vi "FGV ARN Protokoll.vi"(6 "Aktion":T2, 8 "error in (no error)":errorcluster caption="Fehler (Eingang, kein Fehler)", 10 "ResultPictures":T1, 11 "SVGraph Referenz":refnum<vi>) -> (0 "error out":errorcluster caption="Fehler (Ausgang)", 2 "Tabelle Wertänderung":bool, 3 "Tabelle":string[][](array[string]))   [LabVIEW 2020, in "EPA 1065.lvlib" / "ARN Test 1065-305.lvlib"]
uses:
  ARN Test 1065-305.lvlib
  Aktion FGV ARN Protokoll.ctl
  PDF_Interface/PDF Interface Helper/PDFResultPictures.ctl
  Seiten/Gaszuordnung AO/FGV Gaszuordnung Grenzen&Einheit Aktion.ctl
  Aktion FGV ARN Daten.ctl
  Seiten/FT-IR/FGV FT-IR Gasliste Aktionen.ctl
  Sprachverwaltung/FGV Aktion Tabelle zerlegen.ctl
  Cluster PDF.ctl
  Visualisierungs Elemente/String - Ausgabefeld.ctl
  Aktion FGV Protokoll.ctl
  Seiten/Gaszuordnung AO/Gaszuordnung AO.lvlib
  Sprachverwaltung/Sprachverwaltung.lvlib
  Seiten/FT-IR/FT-IR.lvlib
  Linearisierung V2/EPA1065-307/Linearity verification 1065-307.lvlib
  Linearisierung V2/Protokoll/Protokoll.lvlib
  PDF_Interface/PDF Interface Helper/PDF Interface Helper.lvlib
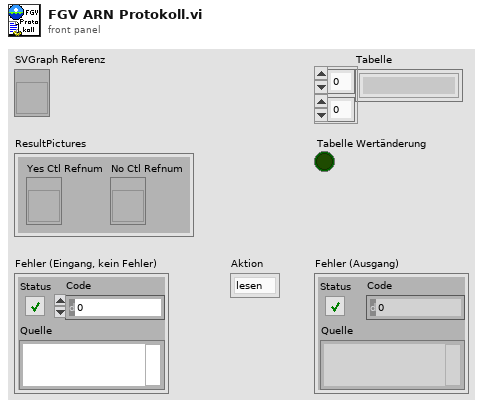
[diagram p1: front panel]
types:
  T1 = typedef "PDF Interface.lvlib/PDF Interface Helper.lvlib/PDFResultPictures.ctl" = cluster{"Yes Ctl Refnum":refnum<vi>, "No Ctl Refnum":refnum<vi>}
  T2 = typedef "EPA 1065.lvlib/ARN Test 1065-305.lvlib/Aktion FGV ARN Protokoll.ctl" = enum16{"lesen", "Tab. schreiben", "Protokoll ausw.", "Protokoll speichern", "Textdatei speichern"}
  T3 = typedef "FT-IR.lvlib/FGV FT-IR Gasliste Aktionen.ctl" = enum16{"lesen", "Gasliste FT-IR", "Gasliste ausgelesen", "laden", "speichern", "löschen"}
  T4 = typedef "EPA 1065.lvlib/ARN Test 1065-305.lvlib/Aktion FGV ARN Daten.ctl" = enum16{"Lesen", "laden", "speichern", "ARN Daten", "Rohdaten", "Rohdaten löschen", "Zeitstempel", "SNR Ergebnis"}
  T5 = typedef "Gaszuordnung AO.lvlib/FGV Gaszuordnung Grenzen&Einheit Aktion.ctl" = enum16{"Lesen", "Schreiben Min", "Schreiben Max", "Laden", "Speichern"}
  T6 = typedef "EPA 1065.lvlib/ARN Test 1065-305.lvlib/Aktion FGV Protokoll.ctl" = enum16{"lesen", "schreiben", "Graph"}
  T7 = typedef "EPA 1065.lvlib/ARN Test 1065-305.lvlib/Cluster PDF.ctl" = cluster{"TAB 1":T8[][], "TAB 2":string[][], "TAB 3":string[][], "Error":bool[]}
  T8 = typedef "String - Ausgabefeld.ctl" = string
  T9 = typedef "Sprachverwaltung.lvlib/FGV Aktion Tabelle zerlegen.ctl" = enum16{"laden", "vereinzeln", "speichern"}
  T10 = enum16{"open", "replace", "create", "open or create", "replace or create", "replace or create with confirmation"}
  T11 = typedef "EPA 1065.lvlib/ARN Test 1065-305.lvlib/Allgemeine Einstellungen.ctl" = cluster{"Bearbeiter:":string, "Analysator":T12, "Komponente:":u16, "Gasflaschen Nr.:":string, "Accuracy":dbl, "Sollwert":dbl, "Modus":T13, "Pfad:":path, "Textname:":string, "CG Aufschaltzeit:":dbl, "Einheit":string, "N2 Aufschaltzeit:":dbl, "Gasflasche":T14, "Konfig Gasflasche":T15}
  T12 = typedef "System Einstellungen V2.lvlib/Analysatoren.ctl" = string
  T13 = typedef "EPA 1065.lvlib/T90 Test 1065-308.lvlib/Modus.ctl" = u16
  T14 = typedef "System Einstellungen V2.lvlib/Gasflasche Auswahl.ctl" = u16
  T15 = typedef "System Einstellungen V2.lvlib/Konfig Gasflasche.ctl" = bool
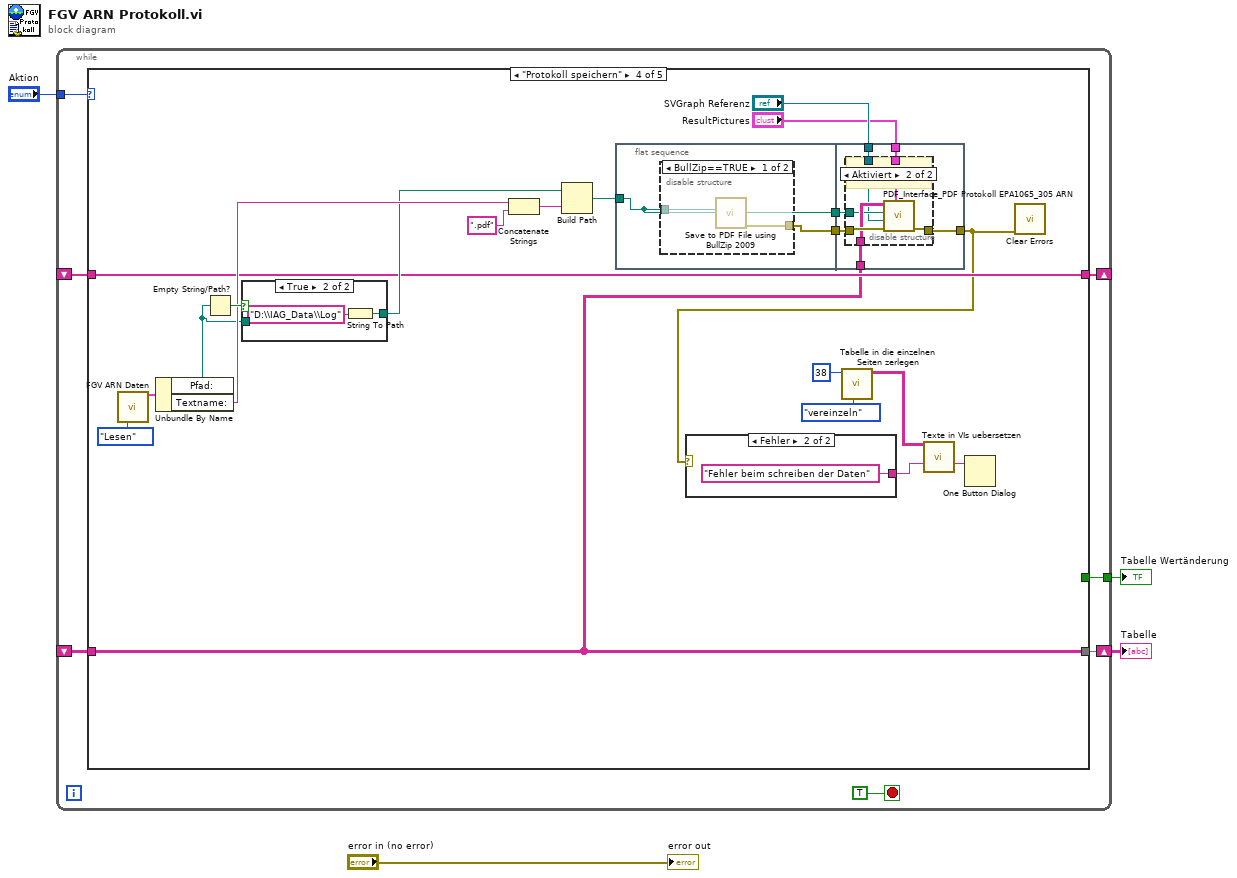
[diagram p0: block diagram]
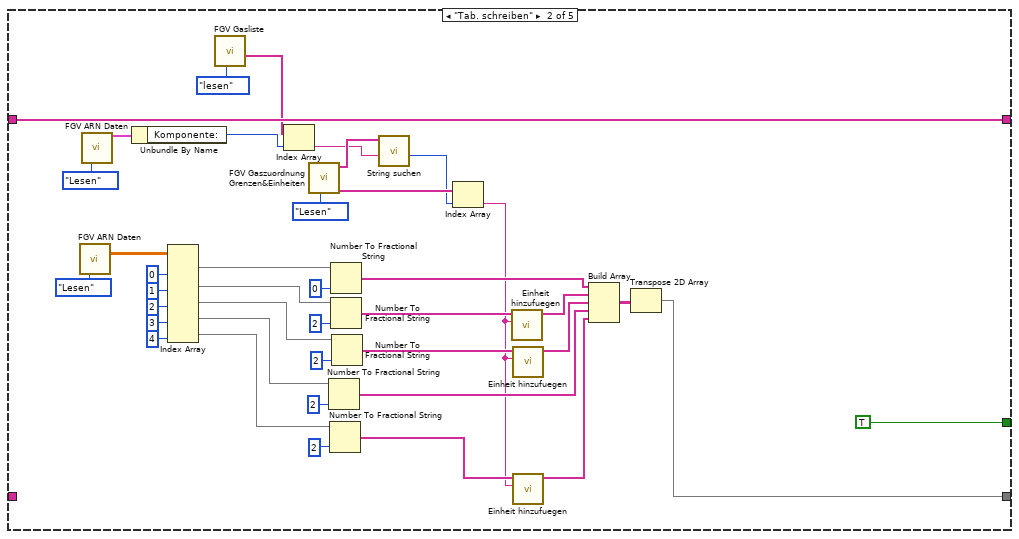
[diagram p3: hidden frame]
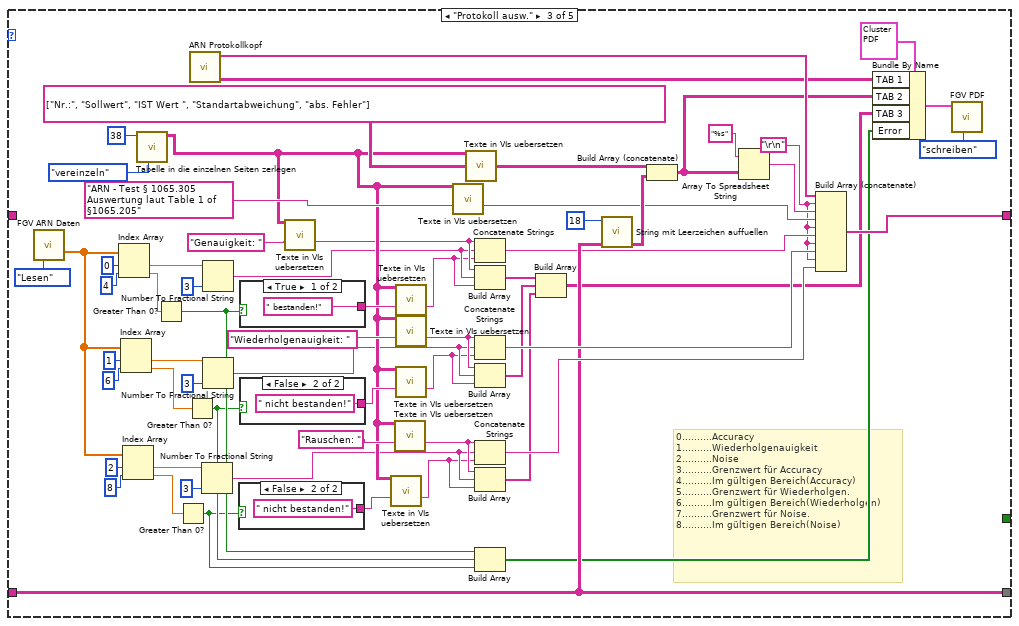
[diagram p4: hidden frame]
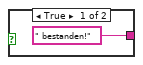
[diagram p5: hidden frame]
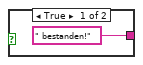
[diagram p6: hidden frame]
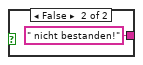
[diagram p7: hidden frame]
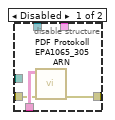
[diagram p9: hidden frame]
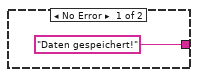
[diagram p11: hidden frame]
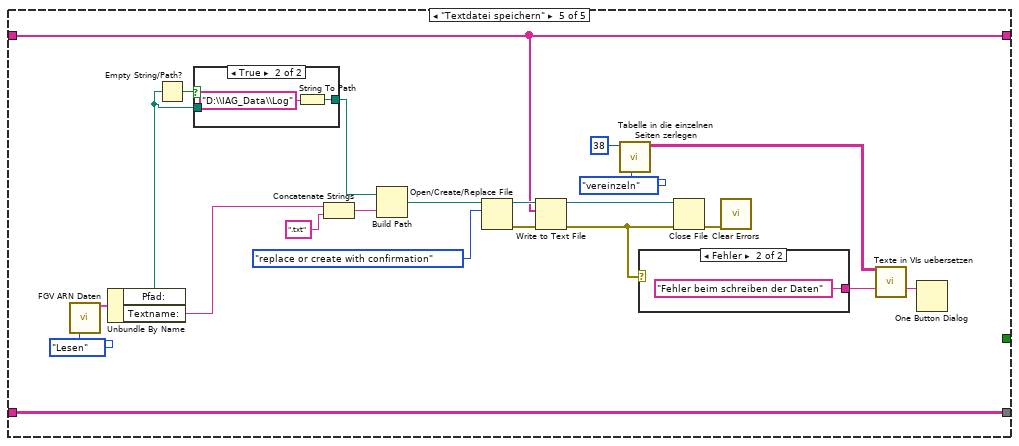
[diagram p12: hidden frame]
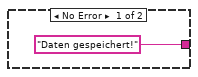
[diagram p14: hidden frame]
diagram:
  n1 = while {
    tunnel: "Aktion" -> [w10]
    shift-right: [w9] -> w3
    shift-left: _ -> [w8]
    shift-right: [w7] -> _
    shift-left: _ -> [w6]
    tunnel: [w5] -> w1
    stop <- TRUE stop-if-true
    n2 = case shown="\"Protokoll speichern\"" w10 {
      tunnel: [w13 w15 w93 w128 w189] -> w9
      tunnel: w8 -> [w13 _ w93 w128 w189]
      tunnel: [w12 w35 w113 w129 w168] -> w7
      tunnel: w6 -> [w12 w35 _ w129 w168]
      tunnel: [_ TRUE _ _ _] -> w5
      frame "lesen", Default {
      }
      frame "Tab. schreiben" {
        n3 = call "FGV ARN Daten.vi"("Aktion"=Aktion_FGV_ARN_Daten."Lesen") -> ("Rohdaten"=w41:sgl[][])  [unwired: 9 in, 5 out]
        n4 = call "FGV ARN Daten.vi"("Aktion"=Aktion_FGV_ARN_Daten."Lesen") -> ("ARN Konfig Daten"=w32:T11)  [unwired: 9 in, 5 out]
        n5 = Unbundle By Name(w32) -> ("Komponente:"=w19:u16)
        n6 = Index Array(array=w41, index (col) #1=0 ("Deaktivierter Index (Spalte)"), index (col) #2=1 ("Index (Spalte)"), index (col) #3=2 ("Index (Spalte)"), index (col) #4=3 ("Index (Spalte)"), index (col) #5=4 ("Index (Spalte)")) -> (element #1=w51:sgl[], element #2=w50:sgl[], element #3=w48:sgl[], element #4=w46:sgl[], element #5=w42:sgl[])  [unwired: 5 in]
        n7 = call "FGV Gasliste.vi"("Aktionen"=FGV_FT-IR_Gasliste_Aktionen."lesen") -> ("Aktuelle Gasliste gesamt"=w20:T8[])  [unwired: 8 in, 2 out]
        n8 = Index Array(array=w20, index=w19) -> (element=w17:T8)
        n9 = call "FGV Gaszuordnung Grenzen&Einheiten.vi"("Aktion"=FGV_Gaszuordnung_Grenzen&Einheit_Aktion."Lesen") -> ("Einheit neu"=w31:string[], "Namen neu"=w18:string[])  [unwired: 2 in, 7 out]
        n10 = Number To Fractional String(number=w46, precision (6)=i16 2 ("Genauigkeit (6)")) -> (F-format string=w29:string[])  [unwired: 2 in]
        n11 = Number To Fractional String(number=w42, precision (6)=i16 2 ("Genauigkeit (6)")) -> (F-format string=w24:string[])  [unwired: 2 in]
        n12 = Number To Fractional String(number=w51, precision (6)=i16 0 ("Genauigkeit (6)")) -> (F-format string=w30:string[])  [unwired: 2 in]
        n13 = Number To Fractional String(number=w50, precision (6)=i16 2 ("Genauigkeit (6)")) -> (F-format string=w28:string[])  [unwired: 2 in]
        n14 = Number To Fractional String(number=w48, precision (6)=i16 2 ("Genauigkeit (6)")) -> (F-format string=w26:string[])  [unwired: 2 in]
        n15 = call "String suchen.vi"("Gasname"=w17, "Such-Namen"=w18) -> ("Index"=w16:i32)  [unwired: 8 in, 1 out]
        n16 = Index Array(array=w31, index=w16) -> (element=w22:string)
        n17 = call "Einheit hinzufuegen.vi"("Einheit"=w22, "Eingang"=w28) -> ("Ausgang"=w27:string[])  [unwired: 9 in]
        n18 = call "Einheit hinzufuegen.vi"("Einheit"=w22, "Eingang"=w26) -> ("Ausgang"=w25:string[])  [unwired: 9 in]
        n19 = call "Einheit hinzufuegen.vi"("Einheit"=w22, "Eingang"=w24) -> ("Ausgang"=w23:string[])  [unwired: 9 in]
        n20 = Build Array(w30, w27, w25, w29, w23) -> (w45:string[][])
        n21 = Transpose 2D Array(2D array=w45) -> (transposed array=w15:string[][])
      }
      frame "Protokoll ausw." {
        w54 = "\r\n"
        # "0..........Accuracy\n1..........Wiederholgenauigkeit\n2..........Noise\n3..........Grenzwert für Accuracy\n4..........Im gültigen Bereich(Accuracy)\n5..........Grenzwert für Wiederholgen.\n6..........Im gültigen Bereich(Wiederholgen)\n7..........Grenzwert für Noise.\n8..........Im gültigen Bereich(Noise)"
        n22 = call "FGV ARN Daten.vi"("Aktion"=Aktion_FGV_ARN_Daten."Lesen") -> ("SNR Ergebnis"=w98:sgl[])  [unwired: 9 in, 5 out]
        n23 = Index Array(array=w98, index #1=0 ("Index"), index #2=4 ("Index")) -> (element #1=w111:sgl, element #2=w108:sgl)
        n24 = Index Array(array=w98, index #1=1 ("Index"), index #2=6 ("Index")) -> (element #1=w101:sgl, element #2=w102:sgl)
        n25 = Index Array(array=w98, index #1=2 ("Index"), index #2=8 ("Index")) -> (element #1=w97:sgl, element #2=w96:sgl)
        n26 = call "Tabelle in die einzelnen Seiten zerlegen.vi"("Aktion"=FGV_Aktion_Tabelle_zerlegen."vereinzeln", "Index (Seite)"=38) -> ("Sprachliste"=w80:string[][])  [unwired: 7 in, 2 out]
        n27 = Greater Than 0?(x=w108) -> (x > 0?=w65:bool)
        n28 = Greater Than 0?(x=w96) -> (x > 0?=w63:bool)
        n29 = Greater Than 0?(x=w102) -> (x > 0?=w64:bool)
        n30 = call "ARN Protokollkopf.vi"() -> ("Angehängtes Array"=w62:T8[][], "Kopfzeile"=w115:string[])  [unwired: 10 in]
        n31 = Number To Fractional String(number=w97, precision (6)=i16 3 ("Genauigkeit (6)")) -> (F-format string=w70:string)  [unwired: 2 in]
        n32 = Number To Fractional String(number=w111, precision (6)=i16 3 ("Genauigkeit (6)")) -> (F-format string=w76:string)  [unwired: 2 in]
        n33 = Number To Fractional String(number=w101, precision (6)=i16 3 ("Genauigkeit (6)")) -> (F-format string=w73:string)  [unwired: 2 in]
        n34 = case shown="False" w63 {
          tunnel: [" bestanden!" " nicht bestanden!"] -> w79
          frame True {
          }
          frame False {
          }
        }
        n35 = case shown="True" w65 {
          tunnel: [" bestanden!" " nicht bestanden!"] -> w84
          frame True {
          }
          frame False {
          }
        }
        n36 = case shown="False" w64 {
          tunnel: [" bestanden!" " nicht bestanden!"] -> w82
          frame True {
          }
          frame False {
          }
        }
        n37 = call "Texte in VIs uebersetzen.vi"("Sprachliste"=w80, "String zum Übersetzen"="Genauigkeit: ") -> ("String zum Übersetzen"=w77:string)  [unwired: 9 in, 4 out]
        n38 = call "Texte in VIs uebersetzen.vi"("Sprachliste"=w80, "String zum Übersetzen"=w79) -> ("String zum Übersetzen"=w69:string)  [unwired: 9 in, 4 out]
        n39 = call "Texte in VIs uebersetzen.vi"("Sprachliste"=w80, "String zum Übersetzen"="Rauschen: ") -> ("String zum Übersetzen"=w71:string)  [unwired: 9 in, 4 out]
        n40 = call "Texte in VIs uebersetzen.vi"("Sprachliste"=w80, "String zum Übersetzen"=w84) -> ("String zum Übersetzen"=w75:string)  [unwired: 9 in, 4 out]
        n41 = call "Texte in VIs uebersetzen.vi"("Sprachliste"=w80, "String zum Übersetzen"="Wiederholgenauigkeit: ") -> ("String zum Übersetzen"=w74:string)  [unwired: 9 in, 4 out]
        n42 = call "Texte in VIs uebersetzen.vi"("Sprachliste"=w80, "String zum Übersetzen"=w82) -> ("String zum Übersetzen"=w72:string)  [unwired: 9 in, 4 out]
        n43 = call "Texte in VIs uebersetzen.vi"("Sprachliste"=w80, "String zum Übersetzen"="ARN - Test § 1065.305 Auswertung laut Table 1 of §1065.205") -> ("String zum Übersetzen"=w86:string)  [unwired: 9 in, 4 out]
        n44 = call "Texte in VIs uebersetzen.vi"("Sprachliste"=w80, "2D String-Array zum Übersetzen"=string[][] [["Nr.:", "Sollwert", "IST Wert ", "Standartabweichung", "abs. Fehler"]]) -> ("2D String-Array zum Übersetzen"=w88:string[][])  [unwired: 9 in, 4 out]
        n45 = Concatenate Strings(w77, w76, w75) -> (w55:string)
        n46 = Build Array(w77, w76, w75) -> (w68:string[])
        n47 = Concatenate Strings(w74, w73, w72) -> (w95:string)
        n48 = Build Array(w74, w73, w72) -> (w67:string[])
        n49 = Concatenate Strings(w71, w70, w69) -> (w94:string)
        n50 = Build Array(w71, w70, w69) -> (w66:string[])
        n51 = Build Array(w65, w64, w63) -> (w59:bool[])
        n52 = Build Array(w68, w67, w66) -> (w60:string[][])
        n53 = call "String mit Leerzeichen auffuellen.vi"("2 Dimension"=w93, "gewünschte Stringgröße"=18) -> ("2 Dimension"=w91:string[][])  [unwired: 8 in, 1 out]
        n54 = Build Array (concatenate)(w88, w91) -> (w61:string[][])
        n55 = Array To Spreadsheet String(array=w61, 3:"%s" ("Format-String")) -> (spreadsheet string=w116:string)  [unwired: 1 in]
        n56 = Build Array (concatenate)(w115, w54, w116, w86, w54, w55, w54, w95, w54, w94) -> (w113:string[])
        n57 = Bundle By Name(cluster=T7 {"TAB 1"=[["ARN-Test §1065.305", ""], ["Datum und Uhrzeit:", ""], ["Bearbeiter:", ""], ["Messgerät:", "FTIR MKS 2030D EPA ready"], ["Komponente:", ""]], "TAB 2"=[], "TAB 3"=[], "Error"=[]} ("Cluster"), "TAB 1"=w62, "TAB 2"=w61, "TAB 3"=w60, "Error"=w59) -> (w56:T7)
        n58 = call "FGV PDF.vi"("Aktion"=Aktion_FGV_Protokoll."schreiben", "Cluster"=w56) -> ()  [unwired: 8 in, 2 out]
      }
      frame "Protokoll speichern" {
        n59 = call "FGV ARN Daten.vi"("Aktion"=Aktion_FGV_ARN_Daten."Lesen") -> ("ARN Konfig Daten"=w133:T11)  [unwired: 9 in, 5 out]
        n60 = Unbundle By Name(w133) -> ("Pfad:"=w130:path, "Textname:"=w132:string)
        n61 = Empty String/Path?(string/path=w130) -> (empty?=w143:bool)
        n62 = case shown="True" w143 {
          tunnel: [w163 w164] -> w131
          tunnel: w130 -> [w163 _]
          frame False {
          }
          frame True {
            n63 = String To Path(string="D:\\IAG_Data\\Log" ("Pfad")) -> (path=w164:path)
          }
        }
        n64 = Concatenate Strings(w132, ".pdf" ("String")) -> (w137:string)
        n65 = Build Path(base path=w131, name or relative path=w137) -> (appended path=w135:path)
        n66 = flat-sequence {
          tunnel: w135 -> [w144]
          tunnel: [w145] -> w127
          tunnel: [w144] -> w125
          tunnel: w128 -> [w153]
          tunnel: w127 -> [w152]
          tunnel: [w151] -> w126
          tunnel: w125 -> [w150]
          tunnel: "SVGraph Referenz" -> [w149]
          tunnel: "ResultPictures" -> [w148]
          frame #0 {
            n67 = disable-structure shown="BullZip==TRUE" {
              disable-tunnel: w144 -> [w147 _]
              disable-tunnel: [w146 _] -> w145
              frame condition #0 {
                n68 = call "Save to PDF File using BullZip 2009.vi"("Save PDF File Path"=w147) -> ("error out"=w146:errorcluster)  [unwired: 10 in]
              }
              frame condition #1 (active) {
              }
            }
          }
          frame #1 {
            n69 = disable-structure shown="Aktiviert" {
              disable-tunnel: w153 -> [w156 w160]
              disable-tunnel: w152 -> [w155 w162]
              disable-tunnel: [w154 w161] -> w151
              disable-tunnel: w150 -> [_ w159]
              disable-tunnel: w149 -> [_ w158]
              disable-tunnel: w148 -> [_ w157]
              frame Disabled {
                n70 = call "PDF Protokoll EPA1065_305 ARN.vi"("error in (no error)"=w155, "Tabelle"=w156) -> ("error out"=w154:errorcluster)  [unwired: 9 in]
              }
              frame Enabled {
                # "#PDF_Interface"
                n71 = call "PDF_Interface_PDF Protokoll EPA1065_305 ARN.vi"("ResultPictures"=w157, "error in (no error)"=w162, "SVGraph Referenz"=w158, "Save PDF File Path"=w159, "Tabelle"=w160) -> ("error out"=w161:errorcluster)  [unwired: 6 in]
              }
            }
          }
        }
        n72 = case shown="Fehler" w126 {
          tunnel: ["Daten gespeichert!" ("String") "Fehler beim schreiben der Daten" ("String")] -> w140
          frame No Error {
          }
          frame Error {
          }
        }
        n73 = call "Tabelle in die einzelnen Seiten zerlegen.vi"("Aktion"=FGV_Aktion_Tabelle_zerlegen."vereinzeln", "Index (Seite)"=38) -> ("Sprachliste"=w141:string[][])  [unwired: 7 in, 2 out]
        n74 = call "Texte in VIs uebersetzen.vi"("Sprachliste"=w141, "String zum Übersetzen"=w140) -> ("String zum Übersetzen"=w139:string)  [unwired: 9 in, 4 out]
        n75 = One Button Dialog(message=w139) -> ()  [unwired: 1 in, 1 out]
        n76 = call <vilib>:"Clear Errors.vi"("error in (no error)"=w126) -> ()  [unwired: 5 in, 2 out]
      }
      frame "Textdatei speichern" {
        n77 = call "FGV ARN Daten.vi"("Aktion"=Aktion_FGV_ARN_Daten."Lesen") -> ("ARN Konfig Daten"=w185:T11)  [unwired: 9 in, 5 out]
        n78 = Unbundle By Name(w185) -> ("Pfad:"=w188:path, "Textname:"=w186:string)
        n79 = Empty String/Path?(string/path=w188) -> (empty?=w181:bool)
        n80 = case shown="True" w181 {
          tunnel: [w190 w191] -> w187
          tunnel: w188 -> [w190 _]
          frame False {
          }
          frame True {
            n81 = String To Path(string="D:\\IAG_Data\\Log" ("Pfad")) -> (path=w191:path)
          }
        }
        n82 = Concatenate Strings(w186, ".txt" ("String")) -> (w176:string)
        n83 = Build Path(base path=w187, name or relative path=w176) -> (appended path=w177:path)
        n84 = Open/Create/Replace File(file path (use dialog)=w177, operation (0:open)=T10."replace or create with confirmation" ("Operation (0:Öffnen)")) -> (refnum out=w174:refnum<file>, error out=w175:errorcluster)  [unwired: 4 in, 1 out]
        n85 = Write to Text File(file (use dialog)=w174, text=w168, error in=w175) -> (refnum out=w179:refnum<file>, error out=w180:errorcluster)  [unwired: 1 in, 1 out]
        n86 = call "Tabelle in die einzelnen Seiten zerlegen.vi"("Aktion"=FGV_Aktion_Tabelle_zerlegen."vereinzeln", "Index (Seite)"=38) -> ("Sprachliste"=w182:string[][])  [unwired: 7 in, 2 out]
        n87 = case shown="Fehler" w180 {
          tunnel: ["Daten gespeichert!" ("String") "Fehler beim schreiben der Daten" ("String")] -> w183
          frame No Error {
          }
          frame Error {
          }
        }
        n88 = Close File(refnum=w179, error in=w180) -> (error out=w178:errorcluster)  [unwired: 1 out]
        n89 = call <vilib>:"Clear Errors.vi"("error in (no error)"=w178) -> ()  [unwired: 5 in, 2 out]
        n90 = call "Texte in VIs uebersetzen.vi"("Sprachliste"=w182, "String zum Übersetzen"=w183) -> ("String zum Übersetzen"=w184:string)  [unwired: 9 in, 4 out]
        n91 = One Button Dialog(message=w184) -> ()  [unwired: 1 in, 1 out]
      }
    }
  }
  "Tabelle" <- w3
  "Tabelle Wertänderung" <- w1
  "error out" <- "error in (no error)"
